vi "midiOutGetNumDevs.vi"(8 "error in":errorcluster, 11 "midi in":refnum<class "midi.lvclass">) -> (0 "error out":errorcluster, 2 "Number of MIDI Output Devices":i32, 3 "midi out":refnum<class "midi.lvclass">)   [LabVIEW 2020, in "midi.lvclass"]
doc: "The midiOutGetNumDevs function retrieves the number of MIDI output devices present in the system.\n\nReturns the number of MIDI output devices. A return value of zero means that there are no devices (not that there is no error)."
uses:
  midi.lvclass
  winmm.dll
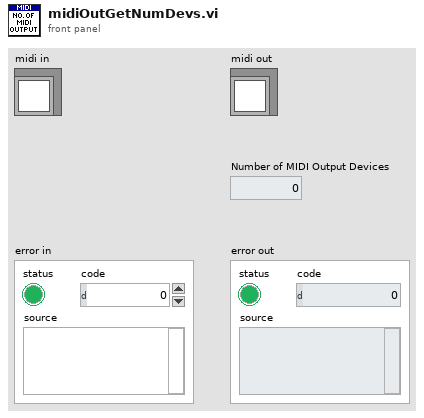
[diagram p1: front panel]
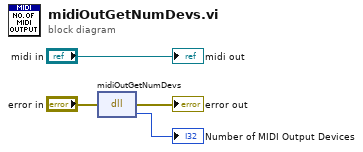
[diagram p0: block diagram]
diagram:
  n1 = dll-call lib="winmm.dll" fn="midiOutGetNumDevs"(error in="error in") -> (error out=→"error out":errorcluster, "NumberOfOutDevices"=→"Number of MIDI Output Devices":i32)  [unwired: 2 in, 1 out]
  "midi out" <- "midi in"
